vi "GLdrv_AMP_TYP.vi"(0 "Connection ID":T2, 7 "CH":i32=1 min=1, 11 "error in (no error)":errorcluster) -> (4 "Connection ID Out":T2, 8 "Type out":T1(ring), 15 "error out":errorcluster)   [LabVIEW 2017, in "GL860_Driver.lvlib"]
doc: "アンプの種類の参照を行います\nOM ：GL800/820用旧端子\nM ：GL240/840/260用端子\nWV ：GL840高精度・高電圧端子\n例）:AMP:CH1:TYP? → :AMP:CH1:TYP M"
uses:
  GL860_Driver.lvlib
  ConnectionID.ctl
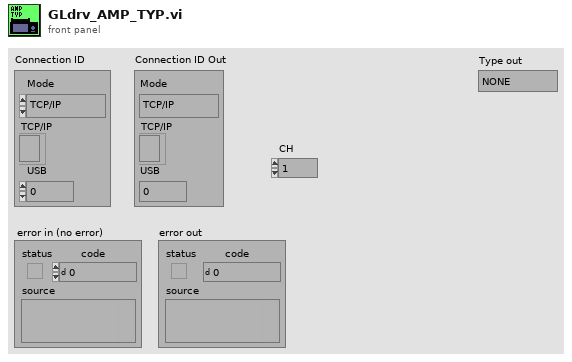
[diagram p1: front panel]
types:
  T1 = enum16{"NONE", "OM", "M", "WV", "NC", "TH", "AT", "VT", "TSR", "LU", "CO2", "AC"}
  T2 = typedef "ConnectionID.ctl" = cluster{"Mode":enum16{"TCP/IP", "USB"}, "TCP/IP":refnum<k5>, "USB":i32}
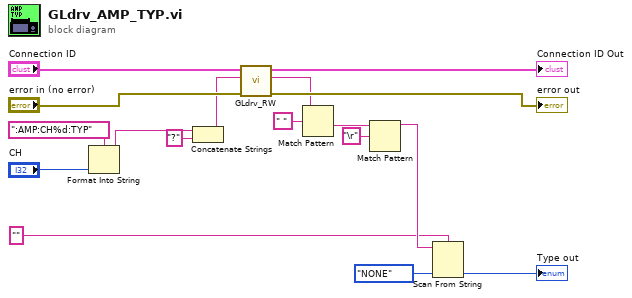
[diagram p0: block diagram]
diagram:
  n1 = Format Into String(format string=":AMP:CH%d:TYP" ("Command"), "CH") -> (resulting string=w13:string)  [unwired: 2 in, 1 out]
  n2 = Concatenate Strings(w13, "?" ("string")) -> (w6:string)
  n3 = call "GLdrv_RW.vi"("error in (no error)"="error in (no error)", "data in"=w6, "Connection ID"="Connection ID") -> ("error out"=→"error out":errorcluster, "data out"=w5:string, "Connection ID Out"=→"Connection ID Out":T2)  [unwired: 4 in, 2 out]
  n4 = Match Pattern(string=w5, regular expression=" " ("search string/char (-)")) -> (after substring=w9:string)  [unwired: 4 out]
  n5 = Match Pattern(string=w9, regular expression="\r") -> (before substring=w7:string)  [unwired: 4 out]
  n6 = Scan From String(format string="" ("Param"), input string=w7, default 1=T1."NONE" ("Type out")) -> (output 1=→"Type out":T1)  [unwired: 2 in, 3 out]
